vi "1.1 Producer Consumer Test 2.vi"() -> ()   [LabVIEW 2018]
uses:
  <vilib>/DAQmx/read.llb/DAQmx Read (Analog 1D Wfm NChan 1Samp).vi
  <vilib>/DAQmx/read.llb/DAQmx Read (Analog 1D Wfm NChan NSamp).vi
  <vilib>/DAQmx/create/channels.llb/DAQmx Create Channel (AI-Voltage-Basic).vi
  <vilib>/DAQmx/configure/timing.llb/DAQmx Timing (Sample Clock).vi
  <vilib>/DAQmx/miscellaneous.llb/DAQmx Fill In Error Info.vi
panel:
  out "Waveform Chart 2":waveform(dbl)[](graph)
  in  "stop":bool
  out "Waveform Chart":waveform(dbl)[](graph)
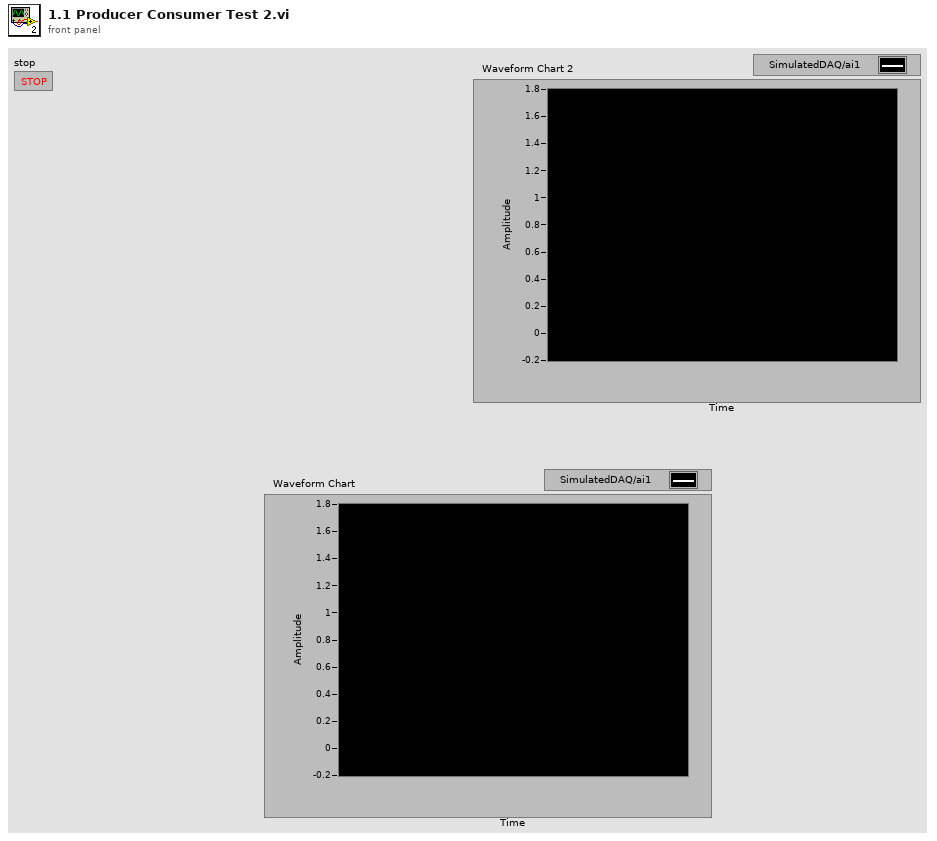
[diagram p1: front panel]
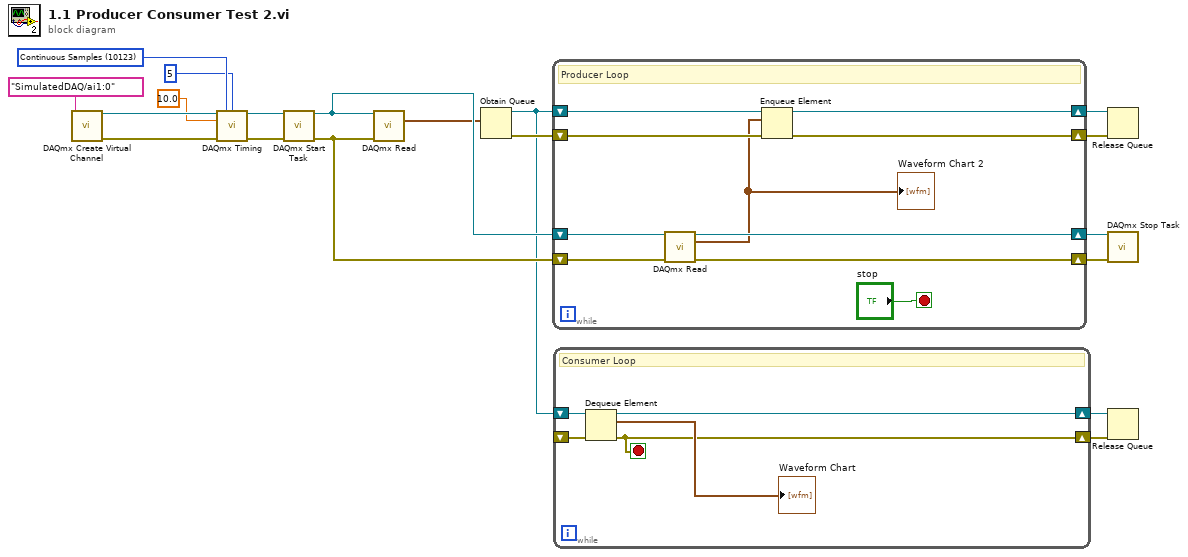
[diagram p0: block diagram]
diagram:
  w15 = 10123 items=["Finite Samples"=10178, "Continuous Samples"=10123, "Hardware Timed Single Point"=12522] ("sample mode")
  n1 = call-poly <vilib>:"DAQmx Create Virtual Channel.vi"("physical channels"=tag "SimulatedDAQ/ai1:0") -> ("task out"=w16:refnum<k21>, "error out"=w17:errorcluster)  [unwired: 13 in]
  n2 = call-poly <vilib>:"DAQmx Timing.vi"("task/channels in"=w16, "sample mode"=w15, "samples per channel"=5, "rate"=10.0, "error in"=w17) -> ("task out"=w18:refnum<k21>, "error out"=w19:errorcluster)  [unwired: 9 in]
  n3 = call <vilib>:"DAQmx Start Task.vi"("task/channels in"=w18, "error in"=w19) -> ("task out"=w12:refnum<k21>, "error out"=w11:errorcluster)  [unwired: 12 in]
  n4 = call-poly <vilib>:"DAQmx Read.vi"("task/channels in"=w12, "error in"=w11) -> ("data"=w10:waveform(dbl)[])  [unwired: 11 in, 2 out]
  n5 = Obtain Queue(element data type=w10) -> (queue out=w4:refnum<queue>, error out=w9:errorcluster)  [unwired: 4 in, 1 out]
  n6 = while {
    shift-right: [w28] -> w6
    shift-left: w12 -> [w22]
    shift-right: [w27] -> w5
    shift-left: w11 -> [w29]
    shift-right: [w23] -> w7
    shift-left: w9 -> [w25]
    shift-right: [w24] -> w8
    shift-left: w4 -> [w26]
    stop <- "stop" stop-if-true
    # "Producer Loop"
    n7 = call-poly <vilib>:"DAQmx Read.vi"("task/channels in"=w22, "error in"=w29) -> ("task out"=w28:refnum<k21>, "data"=w20:waveform(dbl)[], "error out"=w27:errorcluster)  [unwired: 11 in]
    "Waveform Chart 2" <- w20
    n8 = Enqueue Element(queue=w26, element=w20, error in (no error)=w25) -> (queue out=w24:refnum<queue>, error out=w23:errorcluster)  [unwired: 1 in, 1 out]
  }
  n9 = while {
    shift-right: [w33] -> w2
    shift-left: w4 -> [w34]
    shift-right: [w30] -> w1
    shift-left: _ -> [w32]
    stop <- w30 stop-if-true
    # "Consumer Loop"
    n10 = Dequeue Element(queue=w34, error in (no error)=w32) -> (queue out=w33:refnum<queue>, element=→"Waveform Chart":waveform(dbl)[], error out=w30:errorcluster)  [unwired: 1 in, 1 out]
  }
  n11 = Release Queue(queue=w8, error in (no error)=w7) -> ()  [unwired: 1 in, 3 out]
  n12 = call <vilib>:"DAQmx Stop Task.vi"("task/channels in"=w6, "error in"=w5) -> ()  [unwired: 12 in, 2 out]
  n13 = Release Queue(queue=w2, error in (no error)=w1) -> ()  [unwired: 1 in, 3 out]
